vi "手动启动选择对话框.vi"() -> (2 "确定":bool, 3 "输出簇":T2)   [LabVIEW 2016, in "PLC.lvlib"]
uses:
  PLC.lvlib
  <vilib>/Utility/miscctls.llb/LVPointTypeDef.ctl
panel:
  in  "周期运行启动参数":T1
  in  "测试模式":enum16{"正常测试", "集成干预"}(ring)
  in  "取消":bool
  in  "确定":bool
  # "请选择启动参数"
  # "请选择启动模式："
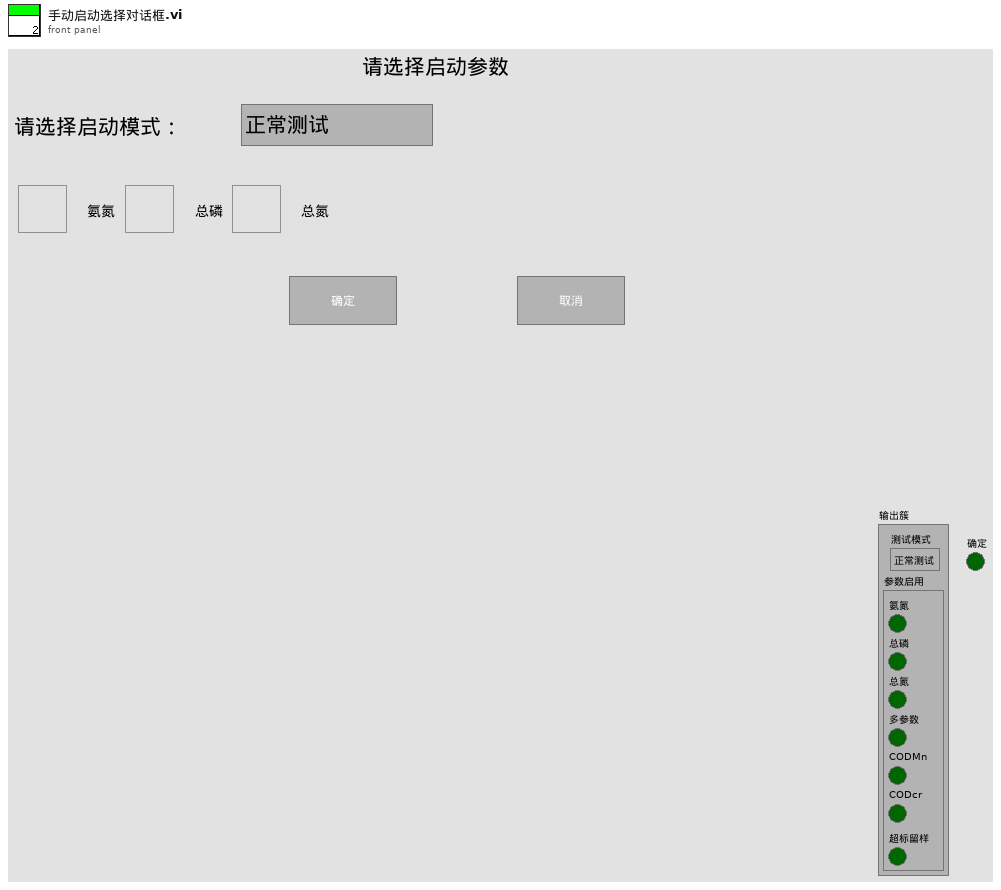
[diagram p1: front panel]
types:
  T1 = cluster{"氨氮":bool, "总磷":bool, "总氮":bool, "多参数":bool, "CODmn":bool, "CODCr":bool, "超标留样":bool}
  T2 = cluster{"测试模式":enum16{"正常测试", "集成干预"}, "参数启用":cluster{"氨氮":bool, "总磷":bool, "总氮":bool, "多参数":bool, "CODMn":bool, "CODcr":bool, "超标留样":bool}}
  T3 = typedef "LVPointTypeDef.ctl" = cluster{"Horizontal":i16, "Vertical":i16}
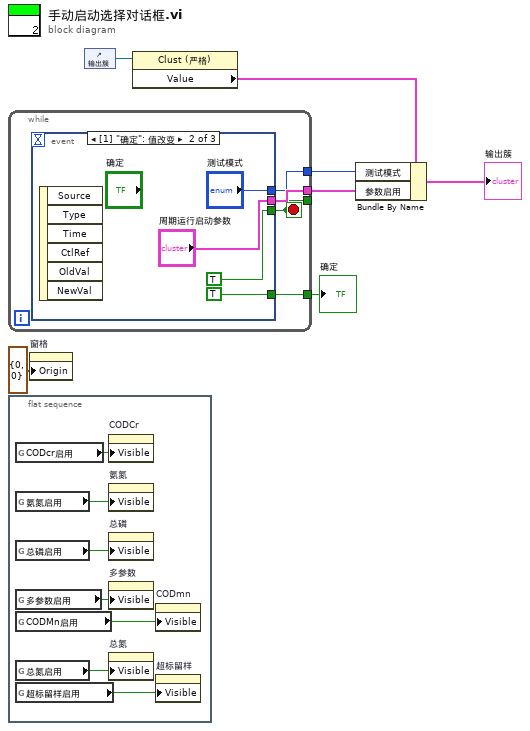
[diagram p0: block diagram]
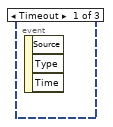
[diagram p2: hidden frame]
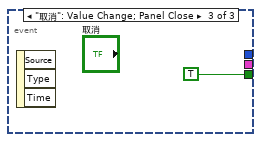
[diagram p3: hidden frame]
diagram:
  n1 = while {
    tunnel: [w11] -> w5
    tunnel: [w10] -> _
    tunnel: [w9] -> w7
    tunnel: [w8] -> w6
    stop <- w10 stop-if-true
    n2 = event shown="[1] \"确定\": 值改变" {
      selector: _ -> [_ _ _]
      dyn-events: _ -> [_ _ _]
      timeout: _ -> [_ _ _]
      tunnel: [_ TRUE TRUE] -> w10
      tunnel: [_ "周期运行启动参数" _] -> w11
      tunnel: [_ TRUE _] -> w9
      tunnel: [_ "测试模式" _] -> w8
      event Timeout {
        n3 = event-data() -> ()  [unwired: 1 in, 3 out]
      }
      event "确定": Value Change {
        n4 = event-data() -> ()  [unwired: 1 in, 6 out]
      }
      event "取消": Value Change; Panel Close {
        n5 = event-data() -> ()  [unwired: 1 in, 3 out]
      }
    }
  }
  "确定" <- w7
  n6 = flat-sequence {
    frame #0 {
      n7 = global read "系统设置全局变量.vi" "CODcr启用"() -> (w19:bool)
      n8 = global read "系统设置全局变量.vi" "氨氮启用"() -> (w23:bool)
      n9 = global read "系统设置全局变量.vi" "总磷启用"() -> (w18:bool)
      n10 = global read "系统设置全局变量.vi" "多参数启用"() -> (w20:bool)
      n11 = global read "系统设置全局变量.vi" "CODMn启用"() -> (w21:bool)
      n12 = global read "系统设置全局变量.vi" "总氮启用"() -> (w22:bool)
      n13 = global read "系统设置全局变量.vi" "超标留样启用"() -> (w17:bool)
      n14 = property on="CODCr" class="Bool (严格)"("Visible"=w19) -> ()  [unwired: 2 in, 2 out]
      n15 = property on="氨氮" class="Bool (严格)"("Visible"=w23) -> ()  [unwired: 2 in, 2 out]
      n16 = property on="总磷" class="Bool (严格)"("Visible"=w18) -> ()  [unwired: 2 in, 2 out]
      n17 = property on="多参数" class="Bool (严格)"("Visible"=w20) -> ()  [unwired: 2 in, 2 out]
      n18 = property on="总氮" class="Bool (严格)"("Visible"=w22) -> ()  [unwired: 2 in, 2 out]
      n19 = property on="CODmn" class="Bool (严格)"("Visible"=w21) -> ()  [unwired: 2 in, 2 out]
      n20 = property on="超标留样" class="Bool (严格)"("Visible"=w17) -> ()  [unwired: 2 in, 2 out]
    }
  }
  n21 = property on="窗格" class="Pane"("Origin"=T3 {"Horizontal"=0, "Vertical"=0} ("原点")) -> ()  [unwired: 2 in, 2 out]
  n22 = control-ref of="输出簇"() -> (w2:refnum<vi>)
  n23 = property class="Clust (严格)"(reference=w2) -> ("Value"=w1:T2)  [unwired: 1 in, 2 out]
  n24 = Bundle By Name(cluster=w1, "测试模式"=w6, "参数启用"=w5) -> (→"输出簇":T2)
